vi "get device ip and port.vi"(0 "variable1":string) -> (1 "port":i32, 2 "port":string, 3 "IP":string)   [LabVIEW 2013]
uses:
  Shared/MySQL/Preset Query Enum.ctl
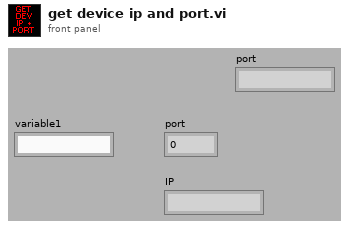
[diagram p1: front panel]
types:
  T1 = typedef "Preset Query Enum.ctl" = enum16{"Get Locations", "Get all IPs and MACs", "Get classes", "Get expt variables to set at scanstart for particular device", "Get expt devices and variables with start values", "Get expt devices and variables (with data to get)", "Get expt devices with data to get", "Get Expt devices and GUIs", "Get all devices basic properties", "Get Virtual Devices Core Info", "Get Expt names", "Get experiment basic properties", "Get experiment alarm variables", "Get MC Ports", "Get device network comm port", "Get devicetype lvclass path", "Get basic device properties", "Get Init Order", "Get all setable variables of a device", "Get device variable aliases", "Get force values of all settable variables", "Get all variables of a devicetype", "Get all variables of a device", "Get plotter details", "Get Saved Scans", "Get Scan Info", "GetGeneralGUIs", "Get expt for plotter", "Get plotter IDs from expt", "Get all devices", "Get all Virtual Devices", "Get all aliases", "Get variable and device info for Virtual Device", "GetItemLocatorIP", "Get IPs for GUIs", "Get DeviceType from Device", "GetLocalPortRange", "GetDevicePresetVariables", "Get Device Configuration", "GetAllPresetNames", "GetAllConfigurationNames", "GetPresetDeviceNames"}
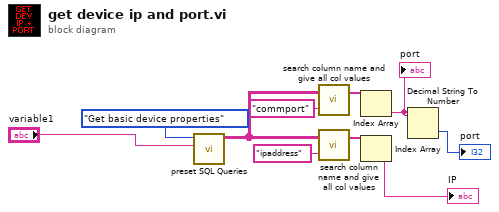
[diagram p0: block diagram]
diagram:
  n1 = call "preset SQL Queries.vi"("Device/Devicetype name\n/Plotter.id/ScanName#"="variable1", "Preset Query"=Preset_Query_Enum."Get basic device properties") -> ("data"=w8:string[][])  [unwired: 7 in, 2 out]
  n2 = call "search column name and give all col values.vi"("column name to get"="commport", "input 2d array"=w8) -> ("column values"=w6:string[])  [unwired: 1 out]
  n3 = call "search column name and give all col values.vi"("column name to get"="ipaddress", "input 2d array"=w8) -> ("column values"=w4:string[])  [unwired: 1 out]
  n4 = Index Array(array=w6) -> (element=w9:string)  [unwired: 1 in]
  "port" <- w9
  n5 = Index Array(array=w4) -> (element=→"IP":string)  [unwired: 1 in]
  n6 = Decimal String To Number(string=w9) -> (number=→"port":i32)  [unwired: 2 in, 1 out]
